vi "MU Acquire 3 Track Mt Sync Data.vi"(6 "AnyThread? (F)":bool, 8 "error in (no error)":errorcluster, 10 "Samples":u64, 11 "MUhandle":u64) -> (0 "error out":errorcluster, 2 "SyncData":T1(array[cluster]), 3 "function return":u32)   [LabVIEW 2017, in "MU_3SL_interface.lvlib"]
uses:
  MU_3SL_interface.lvlib
  lib/MU_3SL_interface.dll
panel:
  in  "SyncData":T2
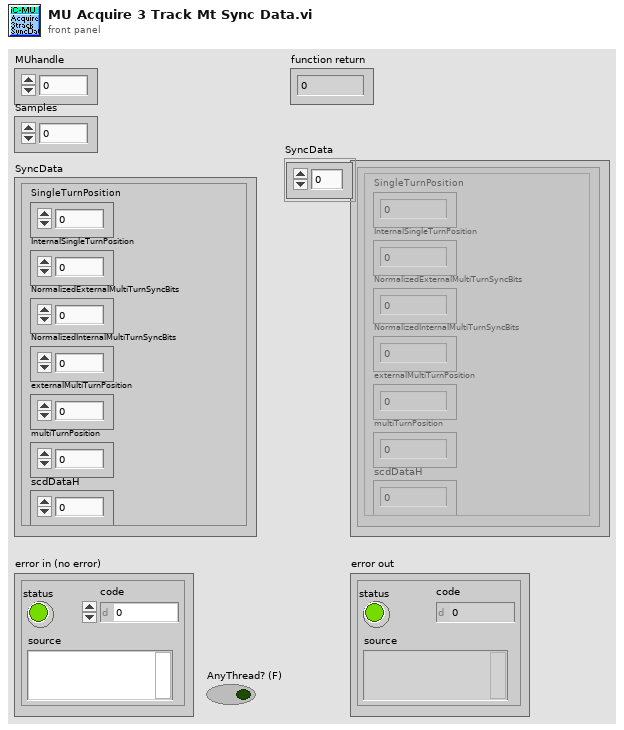
[diagram p1: front panel]
types:
  T1 = cluster{"SingleTurnPosition":u32, "InternalSingleTurnPosition":u32, "NormalizedExternalMultiTurnSyncBits":u32, "NormalizedInternalMultiTurnSyncBits":u32, "externalMultiTurnPosition":u32, "multiTurnPosition":u32, "scdDataH":u64}[]
  T2 = cluster{"SingleTurnPosition":u32, "InternalSingleTurnPosition":u32, "NormalizedExternalMultiTurnSyncBits":u32, "NormalizedInternalMultiTurnSyncBits":u32, "externalMultiTurnPosition":u32, "multiTurnPosition":u32, "scdDataH":u64}
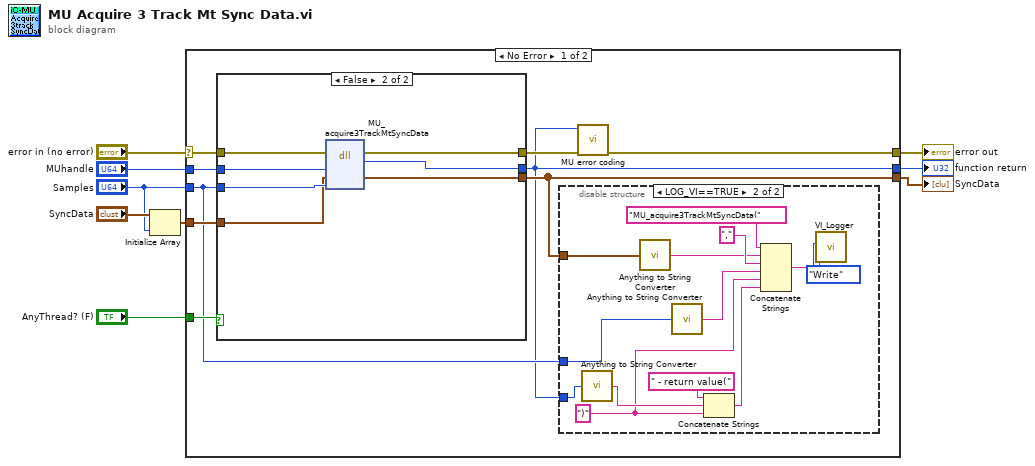
[diagram p0: block diagram]
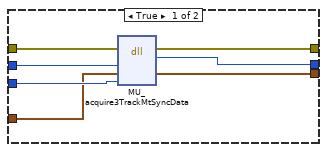
[diagram p2: hidden frame]
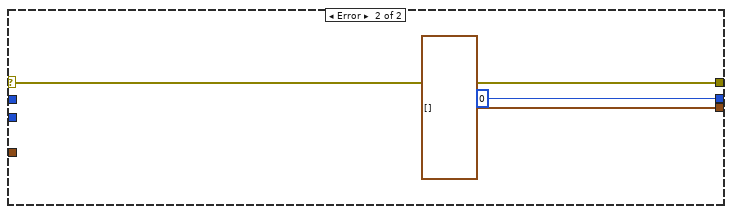
[diagram p4: hidden frame]
diagram:
  n1 = Initialize Array("SyncData", "Samples") -> (w3:T1)
  n2 = case shown="No Error" "error in (no error)" {
    selector: "error in (no error)" -> [w18 w48]
    tunnel: [w10 u32 0 ("function return")] -> w6
    tunnel: [w11 w48] -> w9
    tunnel: "MUhandle" -> [w17 _]
    tunnel: "Samples" -> [w13 _]
    tunnel: w3 -> [w16 _]
    tunnel: [w14 T1 [] ("SyncData")] -> w1
    tunnel: "AnyThread? (F)" -> [w15 _]
    frame No Error {
      n3 = case shown="False" w15 {
        tunnel: w18 -> [w25 w32]
        tunnel: [w24 w31] -> w10
        tunnel: [w23 w30] -> w12
        tunnel: w17 -> [w22 w29]
        tunnel: w13 -> [w21 w28]
        tunnel: w16 -> [w20 w27]
        tunnel: [w19 w26] -> w14
        frame True {
          n4 = dll-call lib="C:/Users/bes/AppData/Roaming/work/mu_9so/icsubmodules/soft_mu_3sl_master/lv_interface/lib/MU_3SL_interface**.*" fn="MU_acquire3TrackMtSyncData"(error in=w25, "MUhandle"=w22, "SyncData"=w20, "Samples"=w21) -> (error out=w23:errorcluster, "function return"=w24:u32, "SyncData"=w19:T1)  [unwired: 4 in, 1 out]
        }
        frame False {
          n5 = dll-call lib="C:/Users/bes/AppData/Roaming/work/mu_9so/icsubmodules/soft_mu_3sl_master/lv_interface/lib/MU_3SL_interface**.*" fn="MU_acquire3TrackMtSyncData"(error in=w32, "MUhandle"=w29, "SyncData"=w27, "Samples"=w28) -> (error out=w30:errorcluster, "function return"=w31:u32, "SyncData"=w26:T1)  [unwired: 4 in, 1 out]
        }
      }
      n6 = disable-structure shown="LOG_VI==TRUE" {
        disable-tunnel: w10 -> [_ w40]
        disable-tunnel: w14 -> [_ w33]
        disable-tunnel: w13 -> [_ w35]
        frame condition #0 {
        }
        frame condition #1 (active) {
          w37 = ")" ("string")
          n7 = call "Anything to String Converter.vi"("anything"=w40) -> ("String"=w39:string)
          n8 = call "Anything to String Converter.vi"("anything"=w33) -> ("String"=w34:string)
          n9 = call "Anything to String Converter.vi"("anything"=w35) -> ("String"=w38:string)
          n10 = Concatenate Strings(" - return value(" ("string"), w39, w37) -> (w36:string)
          n11 = Concatenate Strings("MU_acquire3TrackMtSyncData(" ("Info in"), w34, "," ("string"), w38, w37, w36) -> (w43:string)
          n12 = call "VI_Logger.vi"("Action (Read)"=enum16{"Write", "Read"}."Write", "Info in"=w43) -> ()  [unwired: 8 in, 2 out]
        }
      }
      n13 = call "MU error coding.vi"("error in (no error)"=w12, "function return in"=w10) -> ("error out"=w11:errorcluster)  [unwired: 9 in]
    }
    frame Error {
    }
  }
  "error out" <- w9
  "function return" <- w6
  "SyncData" <- w1
